vi "CRYWindow PIC Project State Change.vi"(9 "sData":string="Save") -> ()   [LabVIEW 2013]
uses:
  CRYProject/CRYProject Editor Global.vi
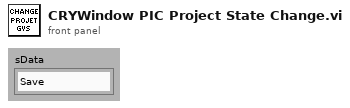
[diagram p1: front panel]
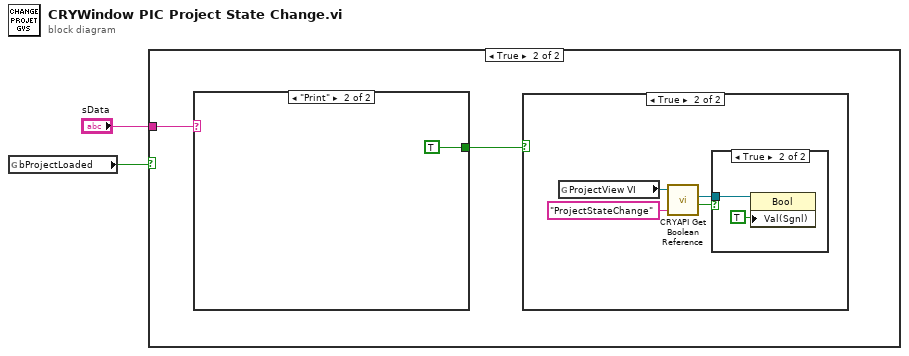
[diagram p0: block diagram]
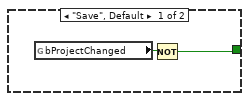
[diagram p5: hidden frame]
diagram:
  n1 = global read "CRYProject Editor Global.vi" "bProjectLoaded"() -> (w2:bool)
  n2 = case shown="True" w2 {
    tunnel: "sData" -> [_ w4]
    frame False {
    }
    frame True {
      n3 = case shown="\"Print\"" w4 {
        tunnel: [w11 TRUE] -> w3
        frame "Save", Default {
          n4 = global read "CRYProject Editor Global.vi" "bProjectChanged"() -> (w12:bool)
          n5 = Not(x=w12) -> (.not. x?=w11:bool)
        }
        frame "Print" {
        }
      }
      n6 = case shown="True" w3 {
        frame False {
        }
        frame True {
          n7 = global read "CRYProject Editor Global.vi" "ProjectView VI"() -> (w8:refnum<vi>)
          n8 = call "CRYAPI Get Boolean Reference.vi"("Label Name"="ProjectStateChange", "VI Refnum"=w8) -> ("Boolean"=w6:bool, "Boolean Ref"=w5:refnum<vi>)  [unwired: 8 out]
          n9 = case shown="True" w6 {
            tunnel: w5 -> [_ w10]
            frame False {
            }
            frame True {
              n10 = property class="Bool"(reference=w10, "Val(Sgnl)"=TRUE) -> ()  [unwired: 1 in, 2 out]
            }
          }
        }
      }
    }
  }
